vi "CorrectALLTDMSFiles.vi"() -> ()   [LabVIEW 2017]
panel:
  out "error out":errorcluster
  out "chemin complet":path
  in  "entrée d'erreur":errorcluster
  in  "chemin":path
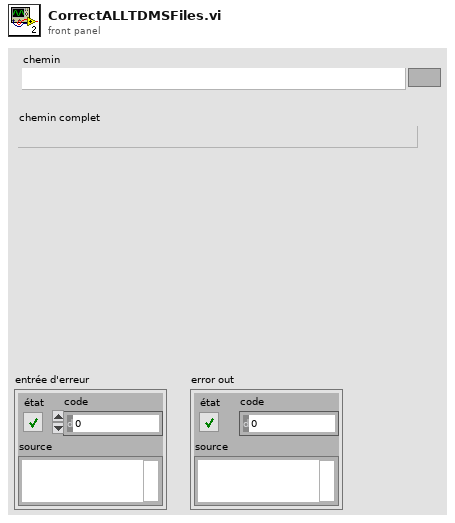
[diagram p1: front panel]
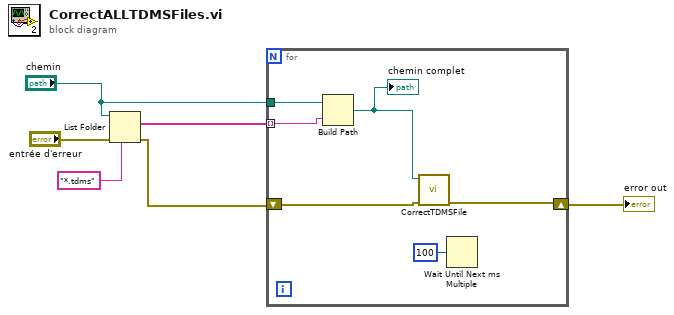
[diagram p0: block diagram]
diagram:
  n1 = List Folder(path="chemin", pattern="*.tdms" ("filtre"), error in="entrée d'erreur") -> (filenames=w4:string[], error out=w5:errorcluster)  [unwired: 1 in, 2 out]
  n2 = for {
    tunnel: w4 -> [w11] mode=indexing
    tunnel: "chemin" -> [w10]
    shift-right: [w8] -> w2
    shift-left: w5 -> [w9]
    n3 = Build Path(base path=w10, name or relative path=w11) -> (appended path=w7:path)
    "chemin complet" <- w7
    n4 = call "CorrectTDMSFile.vi"("entrée d'erreur (pas d'erreur)"=w9, "chemin du fichier"=w7) -> ("sortie d'erreur"=w8:errorcluster)  [unwired: 5 in]
    n5 = Wait Until Next ms Multiple(millisecond multiple=u32 100 ("n millisecondes")) -> ()  [unwired: 1 out]
  }
  "error out" <- w2
